vi "DataGraph_Facade.vi"(0 "Data In":T4, 2 "Display State In":T2, 3 "Container State":T3) -> (6 "Data Out":T4, 7 "Display State Out":T2, 8 "Action":T1)   [LabVIEW 2018, in "DataGraphXControl.xctl"]
uses:
  DataGraphXControl.xctl
  DataGraph_Data.ctl
  <vilib>/_xctls/Container State.ctl
  DataGraph_State.ctl
  <vilib>/_xctls/Action.ctl
  <vilib>/_xctls/XControlSupport.lvlib
panel:
  out "Title_Str":string
  in  "Output_Btn":bool
  in  "List_Btn":bool
  in  "Close_Btn":bool
  in  "Mark_Btn":bool
  out "Info_Listbox":i32(listbox)=-1
  out "Mass_Graph":cluster{"X":dbl[], "Y":dbl[]}[](graph)
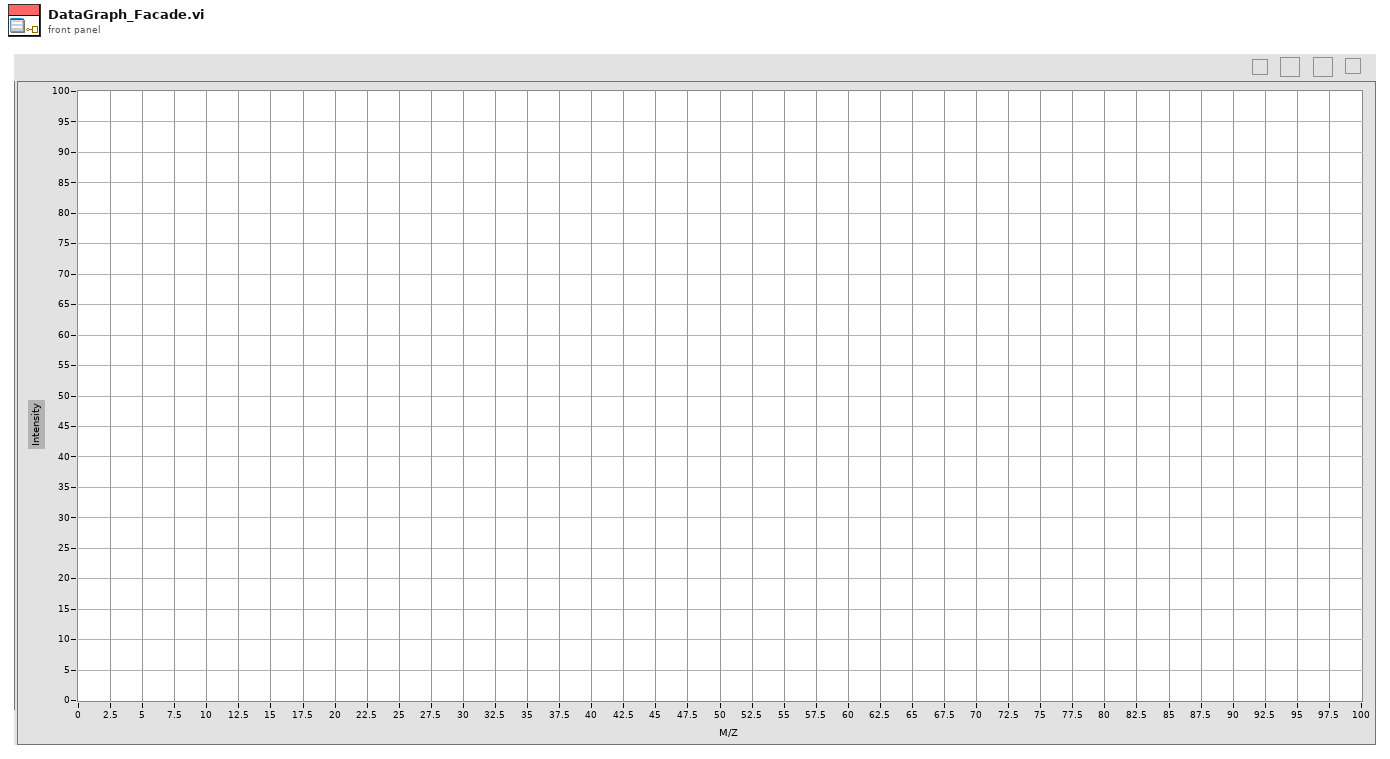
[diagram p1: front panel]
types:
  T1 = typedef "XControlSupport.lvlib/Action.ctl" = cluster{"Data Changed?":bool, "State Changed?":bool, "Action Name":string}
  T2 = typedef "DataGraphXControl.xctl/DataGraph_State.ctl" = cluster{"Mouse State":enum16{"Zoom In", "Select Range"}, "Rectangle X":cluster{"Minimum":dbl, "Maximum":dbl}, "Rectangle Y":cluster{"Minimum":dbl, "Maximum":dbl}, "X Index":cluster{"Minimum":u32, "Maximum":u32}, "FilePath":path, "Allow Index Bool":bool[], "Retangle Enable":bool, "Graph Enable":bool, "Aux Label Enable":bool}
  T3 = typedef "XControlSupport.lvlib/Container State.ctl" = cluster{"Indicator?":bool, "Run Mode?":bool, " Refnum":refnum<vi>}
  T4 = typedef "DataGraphXControl.xctl/DataGraph_Data.ctl" = cluster{"FilePath":path, "Data State":enum16{"Mass", "XIC"}, "Data Plot Names":string[], "DataArray":cluster{"X":dbl[], "Y":dbl[]}[], "Volt Plot Names":string[], "VoltArray":cluster{"X":dbl[], "Y":dbl[]}[], "UserDefine":cluster{"Label":string, "Variant":variant}, "Information":variant}
  T5 = enum16{"No Scaling", "Scale All Objects", "Scale Single Object"}
  T6 = enum8{"Enabled", "Disabled", "Disabled and Grayed Out"}
  T7 = typedef "LVRectTypeDef.ctl" = cluster{"Left":i16, "Top":i16, "Right":i16, "Bottom":i16}
  T8 = typedef "LVPoint32TypeDef.ctl" = cluster{"Horizontal":i32, "Vertical":i32}
  T9 = cluster{"X Scale.Range:Maximum":dbl, "X Scale.Range:Minimum":dbl, "Y Scale.Range:Maximum":dbl, "Y Scale.Range:Minimum":dbl}
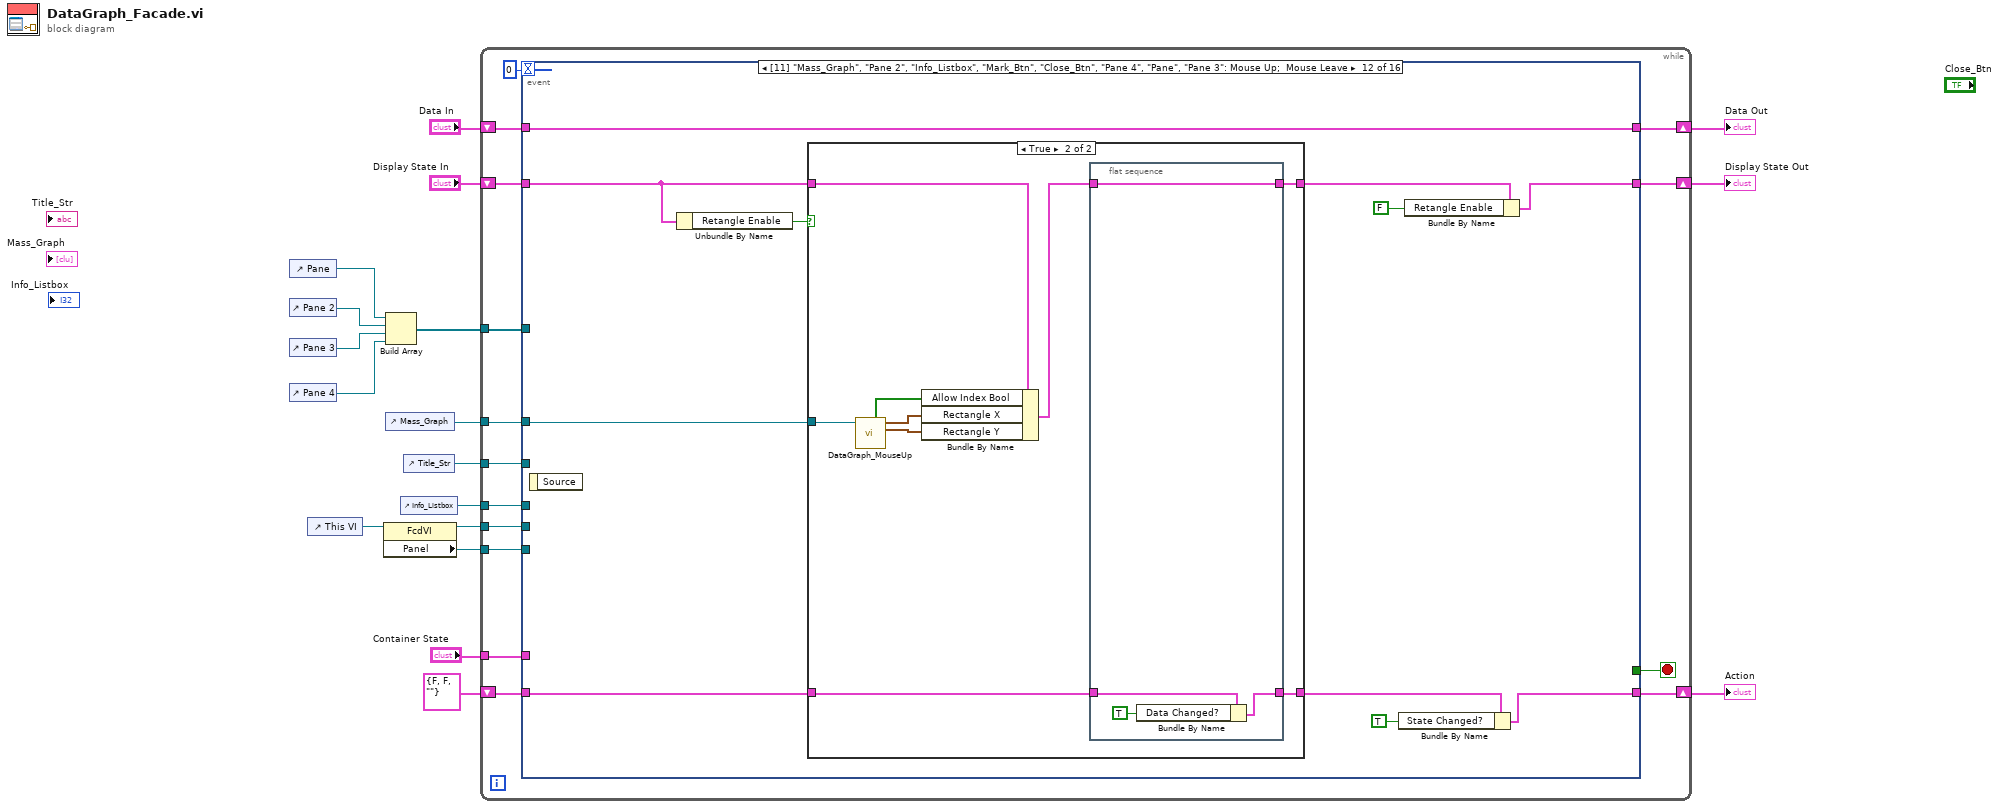
[diagram p0: block diagram]
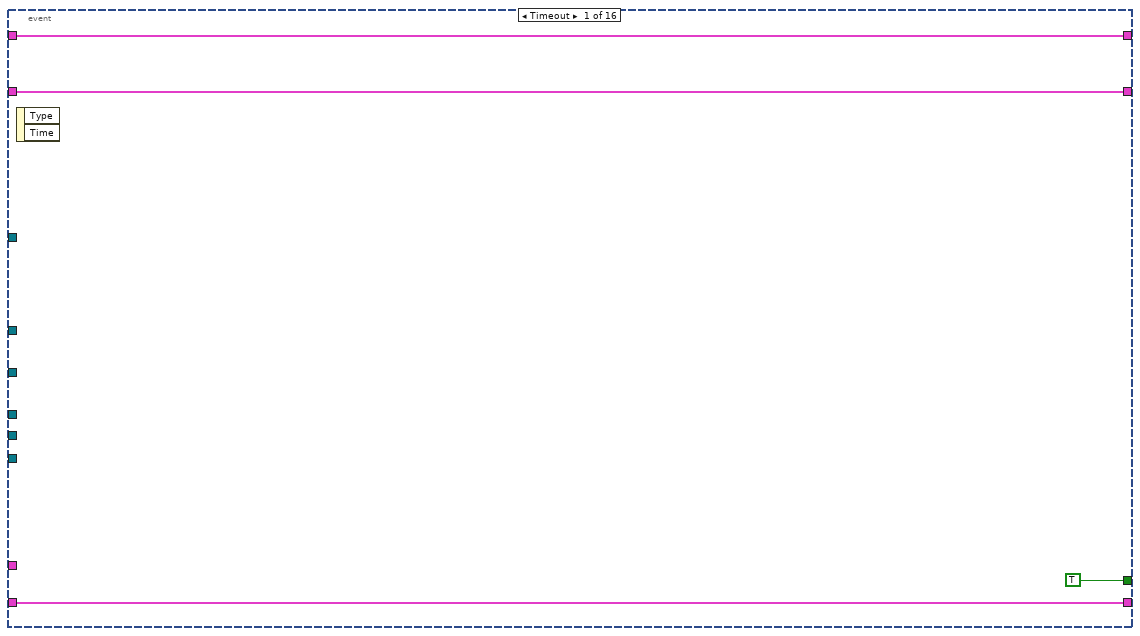
[diagram p2: hidden frame]
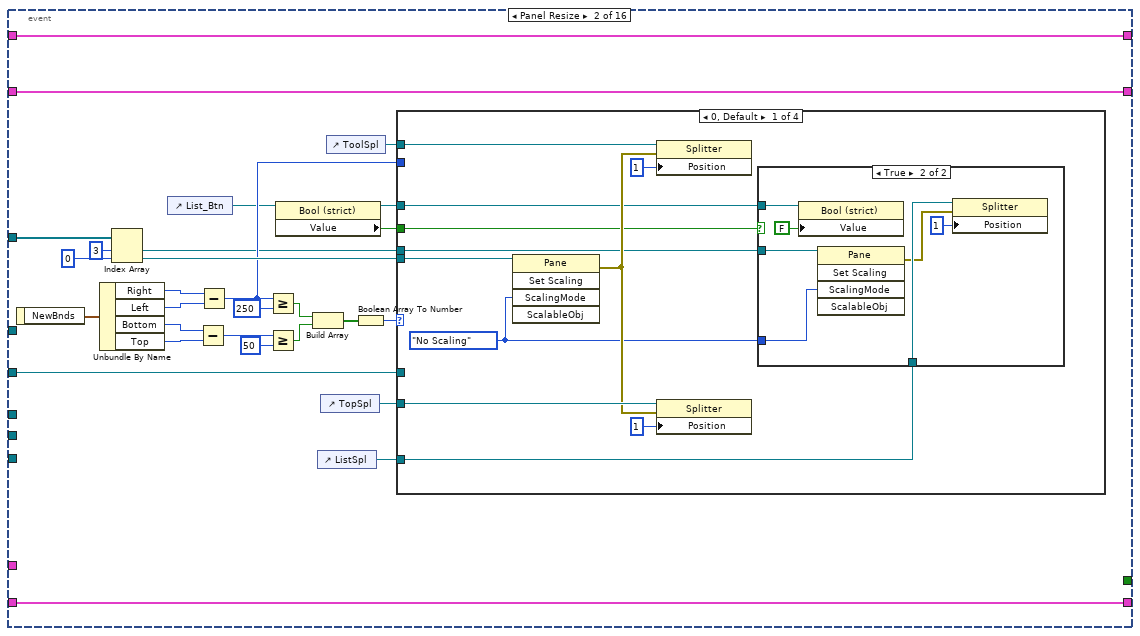
[diagram p3: hidden frame]
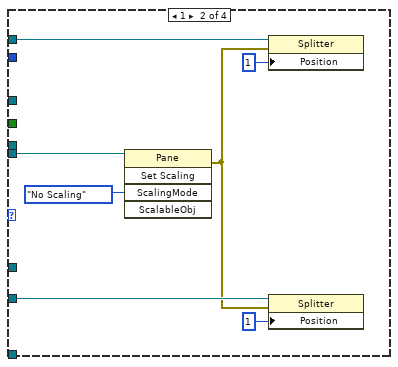
[diagram p5: hidden frame]
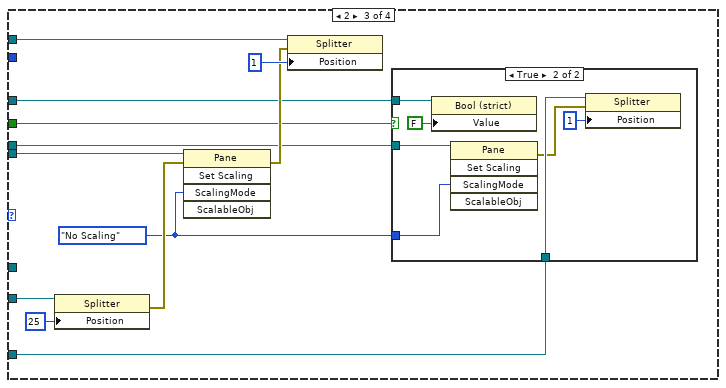
[diagram p6: hidden frame]
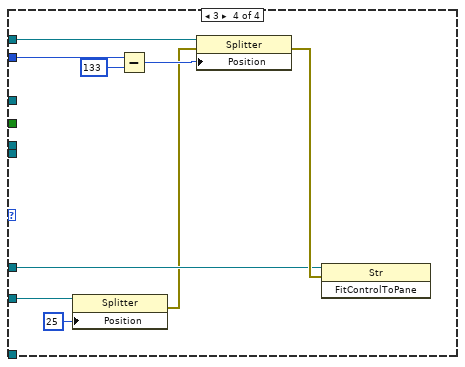
[diagram p8: hidden frame]
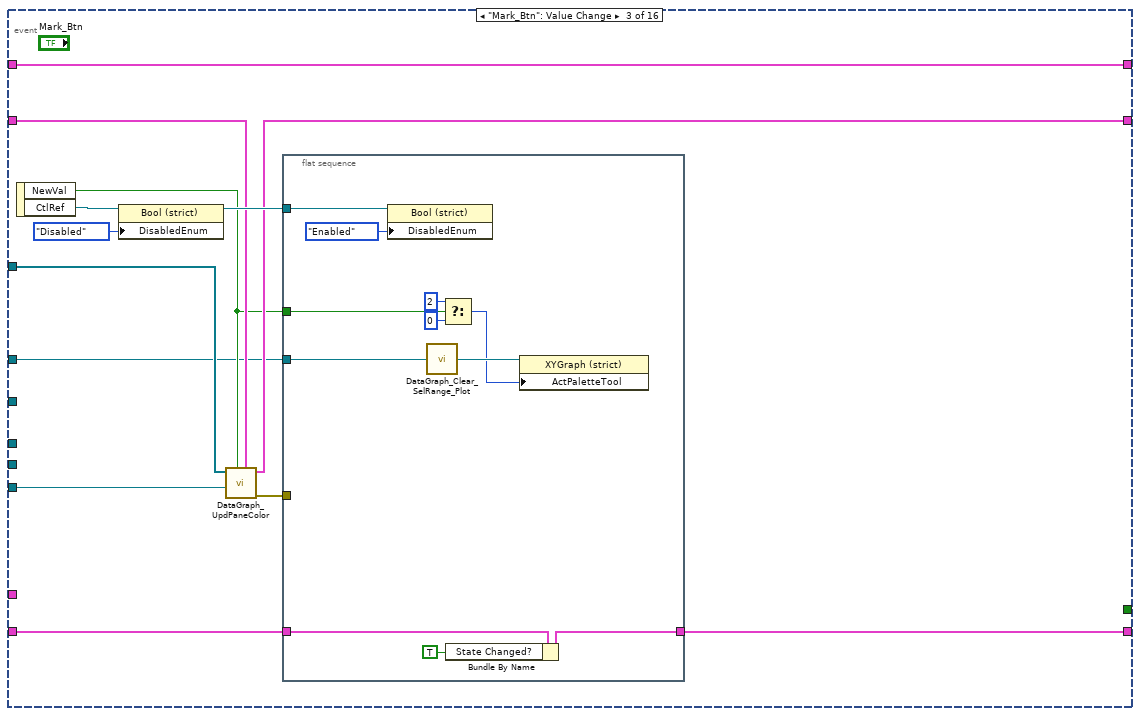
[diagram p9: hidden frame]
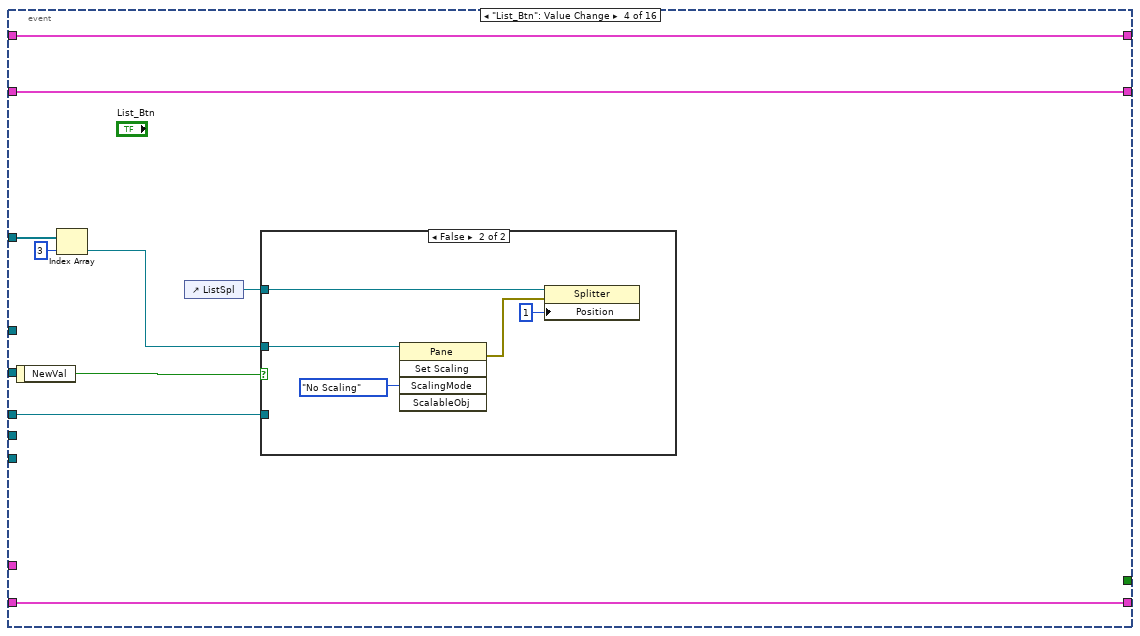
[diagram p10: hidden frame]
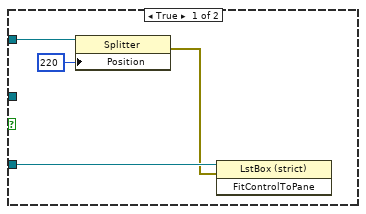
[diagram p11: hidden frame]
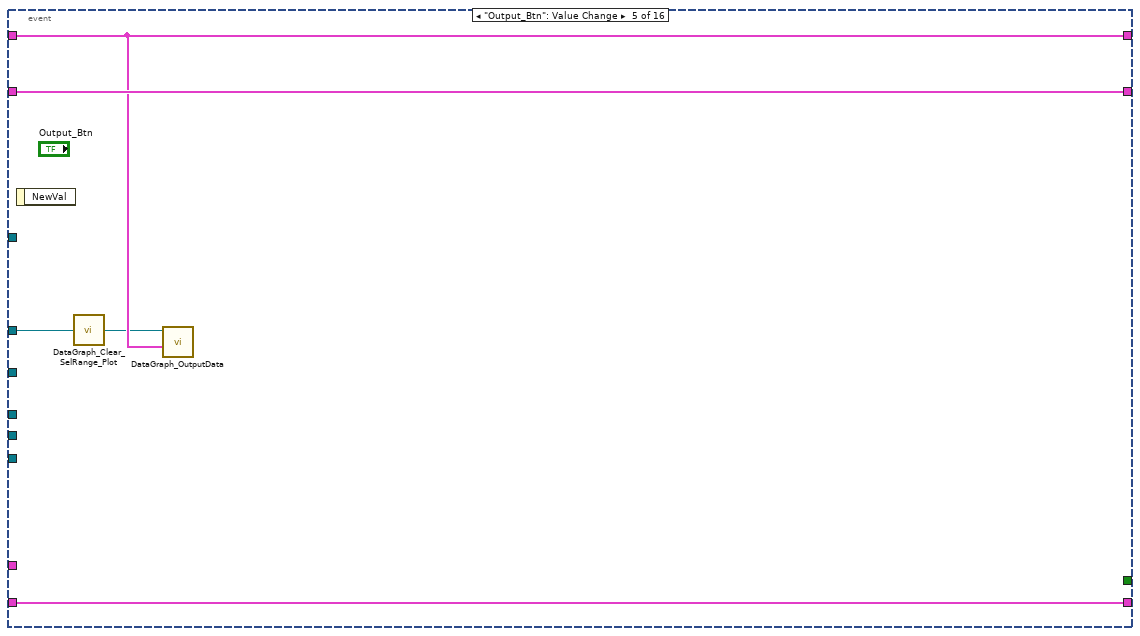
[diagram p12: hidden frame]
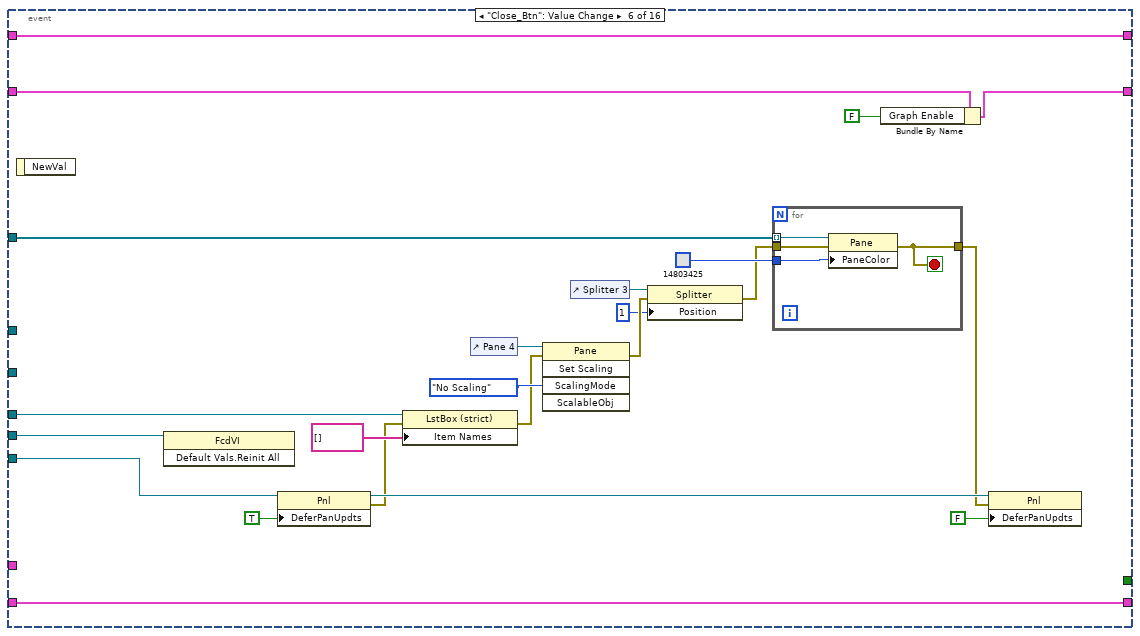
[diagram p13: hidden frame]
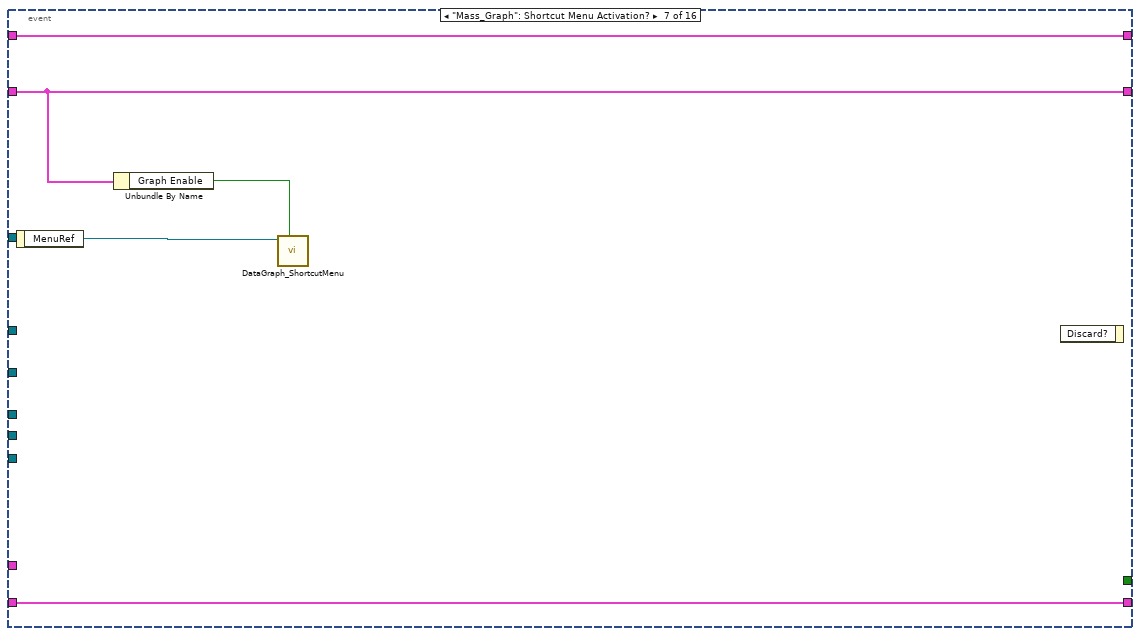
[diagram p14: hidden frame]
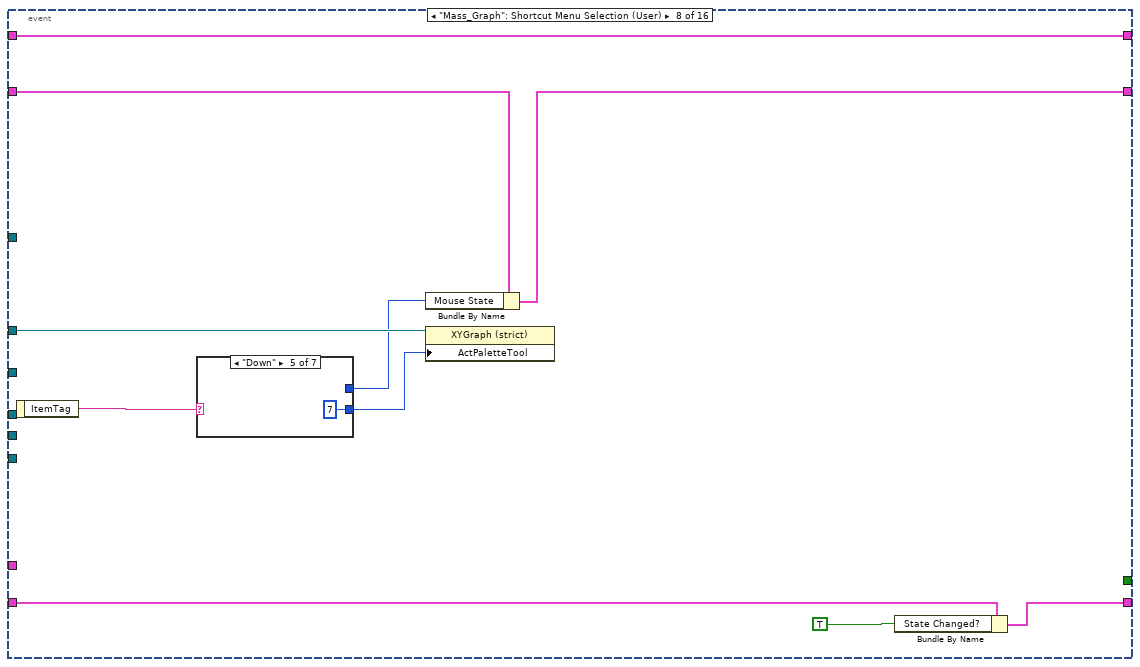
[diagram p15: hidden frame]
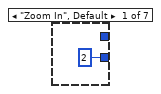
[diagram p16: hidden frame]
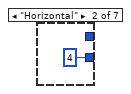
[diagram p17: hidden frame]
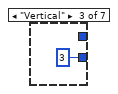
[diagram p18: hidden frame]
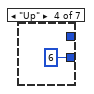
[diagram p19: hidden frame]
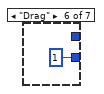
[diagram p20: hidden frame]
diagram:
  n1 = control-ref of="Pane"() -> (w5:refnum<vi>)
  n2 = control-ref of="Pane 2"() -> (w4:refnum<vi>)
  n3 = control-ref of="Pane 3"() -> (w3:refnum<vi>)
  n4 = control-ref of="Pane 4"() -> (w1:refnum<vi>)
  n5 = control-ref of="This VI"() -> (w8:refnum<vi>)
  n6 = property class="FcdVI"(reference=w8) -> (reference out=w6:refnum<vi>, "Panel"=w7:refnum<vi>)  [unwired: 1 in, 1 out]
  n7 = Build Array(w5, w4, w3, w1) -> (w2:refnum<vi>[])
  n8 = control-ref of="Mass_Graph"() -> (w11:refnum<vi>)
  n9 = control-ref of="Info_Listbox"() -> (w9:refnum<vi>)
  n10 = control-ref of="Title_Str"() -> (w10:refnum<vi>)
  n11 = while {
    shift-right: [w32] -> w15
    shift-left: "Display State In" -> [w33]
    tunnel: "Container State" -> [w29]
    shift-right: [w27] -> w18
    shift-left: "Data In" -> [w28]
    shift-right: [w25] -> w13
    shift-left: T1 {"Data Changed?"=FALSE, "State Changed?"=FALSE, "Action Name"=""} ("Action") -> [w26]
    tunnel: w11 -> [w24]
    tunnel: w10 -> [w23]
    tunnel: w9 -> [w22]
    tunnel: w7 -> [w21]
    tunnel: w6 -> [w20]
    tunnel: w2 -> [w19]
    stop <- w31 stop-if-true
    n12 = event shown="[11] \"Mass_Graph\", \"Pane 2\", \"Info_Listbox\", \"Mark_Btn\", \"Close_Btn\", \"Pane 4\", \"Pane\", \"Pane 3\": Mouse Up;  Mouse Leave" {
      selector: _ -> [_ _ _ _ _ _ _ _ _ _ _ _ _ _ _ _]
      dyn-events: _ -> [_ _ _ _ _ _ _ _ _ _ _ _ _ _ _ _]
      timeout: 0 -> [_ _ _ _ _ _ _ _ _ _ _ _ _ _ _ _]
      tunnel: w33 -> [w36 w65 w122 w151 w164 w177 w195 w202 w217 w245 w255 w275 w307 w313 w349 w353]
      tunnel: [w36 w65 w121 w151 w164 w176 w195 w201 w217 w244 w255 w272 w307 w312 w349 w353] -> w32
      tunnel: [TRUE _ _ _ _ _ _ _ _ _ _ _ _ _ _ _] -> w31
      tunnel: w29 -> [_ _ _ _ _ _ _ _ _ _ _ _ _ w321 w350 w354]
      tunnel: w28 -> [w35 w64 w131 w150 w163 w188 w197 w203 w224 w248 w258 w268 w305 w322 w348 w352]
      tunnel: [w35 w64 w131 w150 w163 w188 w197 w203 w224 w248 w258 w268 w305 w322 w348 w352] -> w27
      tunnel: [w34 w63 w129 w146 w165 w187 w196 w204 w223 w242 w257 w270 w306 w314 w347 w351] -> w25
      tunnel: w26 -> [w34 w63 w130 w146 w165 w187 w196 w205 w223 w243 w257 w266 w306 w315 w347 w351]
      tunnel: w24 -> [_ _ w119 _ w162 _ _ w207 w222 w241 _ w274 w302 w311 _ _]
      tunnel: w23 -> [_ w61 _ _ _ _ _ _ _ _ _ _ w303 _ _ _]
      tunnel: w22 -> [_ _ _ w147 _ w185 _ _ _ _ _ _ w304 _ _ _]
      tunnel: w21 -> [_ _ w127 _ _ w174 _ _ _ _ _ _ w296 w318 _ _]
      tunnel: w20 -> [_ _ _ _ _ w186 _ _ _ _ _ _ _ _ _ _]
      tunnel: w19 -> [_ w60 w128 w145 _ w178 _ _ _ _ _ _ _ w317 _ _]
      event Timeout {
        n13 = event-data() -> ()  [unwired: 1 in, 2 out]
      }
      event Panel Resize {
        n14 = event-data() -> ("NewBnds"=w48:T7)  [unwired: 1 in]
        n15 = Unbundle By Name(w48) -> ("Right"=w57:i16, "Left"=w56:i16, "Bottom"=w55:i16, "Top"=w54:i16)
        n16 = Index Array(array=w60, index #1=3 ("index"), index #2=0 ("index")) -> (element #1=w42:refnum<vi>, element #2=w58:refnum<vi>)
        n17 = control-ref of="List_Btn"() -> (w40:refnum<vi>)
        n18 = Subtract(x=w55, y=w54) -> (x-y=w52:i16)
        n19 = Subtract(x=w57, y=w56) -> (x-y=w45:i16)
        n20 = Greater Or Equal?(x=w45, y=i16 250) -> (x >= y?=w50:bool)
        n21 = Greater Or Equal?(x=w52, y=i16 50) -> (x >= y?=w49:bool)
        n22 = property class="Bool (strict)"(reference=w40) -> (reference out=w38:refnum<vi>, "Value"=w39:bool)  [unwired: 1 in, 1 out]
        n23 = Build Array(w50, w49) -> (w47:bool[])
        n24 = control-ref of="ListSpl"() -> (w41:refnum<vi>)
        n25 = control-ref of="TopSpl"() -> (w44:refnum<vi>)
        n26 = control-ref of="ToolSpl"() -> (w62:refnum<vi>)
        n27 = Boolean Array To Number(Boolean array=w47) -> (number=w46:u32)
        n28 = case shown="0, Default" w46 {
          tunnel: w62 -> [w76 w90 w97 w118]
          tunnel: w45 -> [_ _ _ w115]
          tunnel: w61 -> [_ _ _ w113]
          tunnel: w58 -> [w75 w89 w98 _]
          tunnel: w44 -> [w73 w86 w102 w111]
          tunnel: w42 -> [w70 _ w94 _]
          tunnel: w41 -> [w68 _ w93 _]
          tunnel: w39 -> [w67 _ w91 _]
          tunnel: w38 -> [w66 _ w92 _]
          frame 0, Default {
            w69 = T5."No Scaling" ("Scaling Mode")
            n29 = invoke class="Pane" method="Set Scaling"(reference=w75, "ScalingMode"=w69) -> (error out=w71:errorcluster)  [unwired: 3 in, 4 out]
            n30 = property class="Splitter"(reference=w76, error in=w71, "Position"=1 ("Splitter Position")) -> ()  [unwired: 2 out]
            n31 = property class="Splitter"(reference=w73, error in=w71, "Position"=1 ("Splitter Position")) -> ()  [unwired: 2 out]
            n32 = case shown="True" w67 {
              tunnel: w70 -> [_ w83]
              tunnel: w69 -> [_ w82]
              tunnel: w68 -> [_ w81]
              tunnel: w66 -> [_ w78]
              frame False {
              }
              frame True {
                n33 = property class="Bool (strict)"(reference=w78, "Value"=FALSE) -> ()  [unwired: 1 in, 2 out]
                n34 = invoke class="Pane" method="Set Scaling"(reference=w83, "ScalingMode"=w82) -> (error out=w79:errorcluster)  [unwired: 3 in, 4 out]
                n35 = property class="Splitter"(reference=w81, error in=w79, "Position"=1 ("Splitter Position")) -> ()  [unwired: 2 out]
              }
            }
          }
          frame 1 {
            n36 = invoke class="Pane" method="Set Scaling"(reference=w89, "ScalingMode"=T5."No Scaling" ("Scaling Mode")) -> (error out=w84:errorcluster)  [unwired: 3 in, 4 out]
            n37 = property class="Splitter"(reference=w90, error in=w84, "Position"=1 ("Splitter Position")) -> ()  [unwired: 2 out]
            n38 = property class="Splitter"(reference=w86, error in=w84, "Position"=1 ("Splitter Position")) -> ()  [unwired: 2 out]
          }
          frame 2 {
            w95 = T5."No Scaling" ("Scaling Mode")
            n39 = property class="Splitter"(reference=w102, "Position"=25 ("Splitter Position")) -> (error out=w96:errorcluster)  [unwired: 1 in, 1 out]
            n40 = invoke class="Pane" method="Set Scaling"(reference=w98, error in=w96, "ScalingMode"=w95) -> (error out=w99:errorcluster)  [unwired: 2 in, 4 out]
            n41 = property class="Splitter"(reference=w97, error in=w99, "Position"=1 ("Splitter Position")) -> ()  [unwired: 2 out]
            n42 = case shown="True" w91 {
              tunnel: w94 -> [_ w109]
              tunnel: w95 -> [_ w108]
              tunnel: w93 -> [_ w107]
              tunnel: w92 -> [_ w104]
              frame False {
              }
              frame True {
                n43 = property class="Bool (strict)"(reference=w104, "Value"=FALSE) -> ()  [unwired: 1 in, 2 out]
                n44 = invoke class="Pane" method="Set Scaling"(reference=w109, "ScalingMode"=w108) -> (error out=w105:errorcluster)  [unwired: 3 in, 4 out]
                n45 = property class="Splitter"(reference=w107, error in=w105, "Position"=1 ("Splitter Position")) -> ()  [unwired: 2 out]
              }
            }
          }
          frame 3 {
            n46 = property class="Splitter"(reference=w111, "Position"=25 ("Splitter Position")) -> (error out=w110:errorcluster)  [unwired: 1 in, 1 out]
            n47 = Subtract(x=w115, y=i16 133) -> (x-y=w116:i16)
            n48 = property class="Splitter"(reference=w118, error in=w110, "Position"=w116) -> (error out=w114:errorcluster)  [unwired: 1 out]
            n49 = invoke class="Str" method="FitControlToPane"(reference=w113, error in=w114) -> ()  [unwired: 1 in, 3 out]
          }
        }
      }
      event "Mark_Btn": Value Change {
        n50 = event-data() -> ("NewVal"=w120:bool, "CtlRef"=w125:refnum<vi>)  [unwired: 1 in]
        n51 = property class="Bool (strict)"(reference=w125, "DisabledEnum"=T6."Disabled" ("Disabled")) -> (reference out=w123:refnum<vi>)  [unwired: 1 in, 1 out]
        n52 = call "DataGraph_UpdPaneColor.vi"("Display State In"=w122, "Graph Enable"=w120, "Main VI Panel"=w127, "Pane Array"=w128) -> ("error out"=w126:errorcluster, "Display State Out"=w121:T2)  [unwired: 6 in]
        n53 = flat-sequence {
          tunnel: w130 -> [w142]
          tunnel: [w141] -> w129
          tunnel: w126 -> [_]
          tunnel: w123 -> [w138]
          tunnel: w120 -> [w135]
          tunnel: w119 -> [w134]
          frame #0 {
            n54 = property class="Bool (strict)"(reference=w138, "DisabledEnum"=T6."Enabled" ("Disabled")) -> ()  [unwired: 1 in, 2 out]
            n55 = call "DataGraph_Clear_SelRange_Plot.vi"("reference in"=w134) -> ("reference out"=w133:refnum<vi>)
            n56 = Select(t=2 ("Palette:Active Tool"), s=w135, f=0 ("Palette:Active Tool")) -> (s? t:f=w132:i32)
            n57 = Bundle By Name(cluster=w142, "State Changed?"=TRUE ("Data Changed?")) -> (w141:T1)
            n58 = property class="XYGraph (strict)"(reference=w133, "ActPaletteTool"=w132) -> ()  [unwired: 1 in, 2 out]
          }
        }
      }
      event "List_Btn": Value Change {
        n59 = event-data() -> ("NewVal"=w149:bool)  [unwired: 1 in]
        n60 = Index Array(array=w145, index=3) -> (element=w143:refnum<vi>)
        n61 = control-ref of="ListSpl"() -> (w148:refnum<vi>)
        n62 = case shown="False" w149 {
          tunnel: w148 -> [w154 w157]
          tunnel: w143 -> [_ w156]
          tunnel: w147 -> [w153 _]
          frame True {
            n63 = property class="Splitter"(reference=w154, "Position"=220 ("Splitter Position")) -> (error out=w152:errorcluster)  [unwired: 1 in, 1 out]
            n64 = invoke class="LstBox (strict)" method="FitControlToPane"(reference=w153, error in=w152) -> ()  [unwired: 1 in, 3 out]
          }
          frame False {
            n65 = invoke class="Pane" method="Set Scaling"(reference=w156, "ScalingMode"=T5."No Scaling" ("Scaling Mode")) -> (error out=w158:errorcluster)  [unwired: 3 in, 4 out]
            n66 = property class="Splitter"(reference=w157, error in=w158, "Position"=1 ("Splitter Position")) -> ()  [unwired: 2 out]
          }
        }
      }
      event "Output_Btn": Value Change {
        n67 = event-data() -> ()  [unwired: 1 in, 1 out]
        n68 = call "DataGraph_Clear_SelRange_Plot.vi"("reference in"=w162) -> ("reference out"=w161:refnum<vi>)
        n69 = call "DataGraph_OutputData.vi"("Data In"=w163, "Mass_Graph"=w161) -> ()  [unwired: 10 in]
      }
      event "Close_Btn": Value Change {
        n70 = event-data() -> ()  [unwired: 1 in, 1 out]
        n71 = invoke class="FcdVI" method="Default Vals.Reinit All"(reference=w186) -> ()  [unwired: 2 in, 3 out]
        n72 = property class="Pnl"(reference=w174, "DeferPanUpdts"=TRUE ("Defer Panel Updates")) -> (reference out=w182:refnum<vi>, error out=w167:errorcluster)  [unwired: 1 in]
        n73 = property class="LstBox (strict)"(reference=w185, error in=w167, "Item Names"=string[] []) -> (error out=w166:errorcluster)  [unwired: 1 out]
        n74 = control-ref of="Pane 4"() -> (w173:refnum<vi>)
        n75 = invoke class="Pane" method="Set Scaling"(reference=w173, error in=w166, "ScalingMode"=T5."No Scaling" ("Scaling Mode")) -> (error out=w171:errorcluster)  [unwired: 2 in, 4 out]
        n76 = control-ref of="Splitter 3"() -> (w172:refnum<vi>)
        n77 = property class="Splitter"(reference=w172, error in=w171, "Position"=1 ("Splitter Position")) -> (error out=w168:errorcluster)  [unwired: 1 out]
        n78 = for {
          tunnel: w178 -> [w192] mode=indexing
          tunnel: u32 14803425 -> [w191]
          tunnel: w168 -> [w190]
          tunnel: [w189] -> w179
          stop <- w189 stop-if-true
          n79 = property class="Pane"(reference=w192, error in=w190, "PaneColor"=w191) -> (error out=w189:errorcluster)  [unwired: 1 out]
        }
        n80 = Bundle By Name(cluster=w177, "Graph Enable"=FALSE) -> (w176:T2)
        n81 = property class="Pnl"(reference=w182, error in=w179, "DeferPanUpdts"=FALSE ("Defer Panel Updates")) -> ()  [unwired: 2 out]
      }
      event "Mass_Graph": Shortcut Menu Activation? {
        n82 = event-data() -> ("MenuRef"=w193:refnum<k9>)  [unwired: 1 in]
        n83 = Unbundle By Name(w195) -> ("Graph Enable"=w194:bool)
        n84 = call "DataGraph_ShortcutMenu.vi"("ShortCut Menu Enable"=w194, "menu reference"=w193) -> ()  [unwired: 8 in, 2 out]
        n85 = event-data() -> ()  [unwired: 2 in, 1 out]
      }
      event "Mass_Graph": Shortcut Menu Selection (User) {
        n86 = event-data() -> ("ItemTag"=w200:string)  [unwired: 1 in]
        n87 = case shown="\"Down\"" w200 {
          tunnel: [2 ("Palette:Active Tool") 4 ("Palette:Active Tool") 3 ("Palette:Active Tool") 6 ("Palette:Active Tool") 7 ("Palette:Active Tool") 1 ("Palette:Active Tool") 0 ("Palette:Active Tool")] -> w199
          tunnel: [_ _ _ _ _ _ enum16{"Zoom In", "Select Range"}."Select Range" ("Mouse State")] -> w198
          frame "Zoom In", Default {
          }
          frame "Horizontal" {
          }
          frame "Vertical" {
          }
          frame "Up" {
          }
          frame "Down" {
          }
          frame "Drag" {
          }
          frame "Select Range" {
          }
        }
        n88 = Bundle By Name(cluster=w202, "Mouse State"=w198) -> (w201:T2)
        n89 = property class="XYGraph (strict)"(reference=w207, "ActPaletteTool"=w199) -> ()  [unwired: 1 in, 2 out]
        n90 = Bundle By Name(cluster=w205, "State Changed?"=TRUE ("Data Changed?")) -> (w204:T1)
      }
      event "Mass_Graph": Mouse Down? {
        n91 = event-data() -> ("Button"=w221:u16, "Mods.Double Click"=w220:bool)  [unwired: 1 in]
        n92 = Unbundle By Name(w217) -> ("Mouse State"=w219:enum16{"Zoom In", "Select Range"})
        n93 = Equal?(x=w219, y=enum16{"Zoom In", "Select Range"}."Select Range") -> (x = y?=w216:bool)
        n94 = case shown="False" w216 {
          tunnel: w222 -> [w230 _]
          tunnel: w221 -> [w229 _]
          tunnel: w220 -> [w226 _]
          frame False {
            n95 = Equal?(x=u16 1, y=w229) -> (x = y?=w227:bool)
            n96 = And(x=w227, y=w226) -> (x .and. y?=w225:bool)
            n97 = case shown="True" w225 {
              tunnel: w230 -> [_ w231]
              frame False {
              }
              frame True {
                n98 = property class="XYGraph (strict)"(reference=w231, "ActPaletteTool"=5 ("Palette:Active Tool")) -> ()  [unwired: 1 in, 2 out]
              }
            }
          }
          frame True {
          }
        }
        n99 = event-data() -> ()  [unwired: 2 in, 1 out]
      }
      event "Mass_Graph": Mouse Down {
        n100 = event-data() -> ("Button"=w247:u16, "Coords"=w240:T8)  [unwired: 1 in]
        n101 = Unbundle By Name(w245) -> ("Mouse State"=w239:enum16{"Zoom In", "Select Range"})
        n102 = Equal?(x=u16 1, y=w247) -> (x = y?=w235:bool)
        n103 = Equal?(x=w239, y=enum16{"Zoom In", "Select Range"}."Select Range") -> (x = y?=w234:bool)
        n104 = And(x=w234, y=w235) -> (x .and. y?=w233:bool)
        n105 = case shown="True" w233 {
          selector: w233 -> [w249 w253]
          tunnel: w241 -> [_ w252]
          tunnel: [w249 w253] -> w237
          tunnel: w240 -> [_ w251]
          frame False {
          }
          frame True {
            n106 = call "DataGraph_MouseInit.vi"("State"=enum16{"Read", "Write"}."Write", "Point32"=w251, "Mass_Graph"=w252) -> ()  [unwired: 5 in, 4 out]
          }
        }
        n107 = Bundle By Name(cluster=w243, "State Changed?"=TRUE) -> (w242:T1)
        n108 = Bundle By Name(cluster=w245, "Retangle Enable"=w237) -> (w244:T2)
      }
      event "Mass_Graph": Mouse Move {
        n109 = event-data() -> ("Coords"=w256:T8)  [unwired: 1 in]
        n110 = Unbundle By Name(w255) -> ("Retangle Enable"=w254:bool)
        n111 = case shown="True" w254 {
          tunnel: w256 -> [_ w260]
          frame False {
          }
          frame True {
            n112 = call "DataGraph_MouseInit.vi"("State"=enum16{"Read", "Write"}."Read") -> ("error out"=w264:errorcluster, "Point32"=w262:T8, "reference out"=w263:refnum<vi>, "Boundary"=w259:T9)  [unwired: 7 in]
            n113 = call "DataGraph_MouseMove.vi"("Boundary"=w259, "error in (no error)"=w264, "Point32"=w260, "Raw Coords"=w262, "Mass_Graph"=w263) -> ()  [unwired: 6 in, 1 out]
          }
        }
      }
      event "Mass_Graph", "Info_Listbox", "Mark_Btn", "Close_Btn": Mouse Up; Mouse Leave {
        n114 = event-data() -> ()  [unwired: 1 in, 1 out]
        n115 = Unbundle By Name(w275) -> ("Retangle Enable"=w273:bool)
        n116 = case shown="True" w273 {
          tunnel: w275 -> [w277 w286]
          tunnel: w274 -> [_ w285]
          tunnel: [w277 w282] -> w269
          tunnel: w266 -> [w276 w284]
          tunnel: [w276 w283] -> w265
          frame False {
          }
          frame True {
            n117 = call "DataGraph_MouseUp.vi"("Mass_Graph"=w285) -> ("Rectangle Y"=w279:cluster{"Minimum":dbl, "Maximum":dbl}, "Rectangle X"=w280:cluster{"Minimum":dbl, "Maximum":dbl}, "Allow Index Bool"=w278:bool[])  [unwired: 7 in, 1 out]
            n118 = Bundle By Name(cluster=w286, "Allow Index Bool"=w278, "Rectangle X"=w280, "Rectangle Y"=w279) -> (w281:T2)
            n119 = flat-sequence {
              tunnel: w284 -> [w290]
              tunnel: [w288] -> w283
              tunnel: [w287] -> w282
              tunnel: w281 -> [w287]
              frame #0 {
                n120 = Bundle By Name(cluster=w290, "Data Changed?"=TRUE) -> (w288:T1)
              }
            }
          }
        }
        n121 = Bundle By Name(cluster=w265, "State Changed?"=TRUE) -> (w270:T1)
        n122 = Bundle By Name(cluster=w269, "Retangle Enable"=FALSE) -> (w272:T2)
      }
      event Data Change {
        n123 = event-data() -> ()  [unwired: 1 in, 1 out]
        n124 = property class="Pnl"(reference=w296, "DeferPanUpdts"=TRUE ("Defer Panel Updates")) -> (reference out=w292:refnum<vi>, error out=w294:errorcluster)  [unwired: 1 in]
        n125 = call "DataGraph_UpdateInterface.vi"("Data In"=w305, "error in (no error)"=w294, "Info_Listbox"=w304, "Title_Str"=w303, "Mass_Graph"=w302) -> ("error out"=w301:errorcluster)  [unwired: 6 in]
        n126 = property class="XYGraph (strict)"(reference=w302, error in=w301, "ActPaletteTool"=0 ("Palette:Active Tool")) -> (reference out=w299:refnum<vi>, error out=w298:errorcluster)
        n127 = property class="XYGraph (strict)"(reference=w299, error in=w298, "ActPaletteTool"=5 ("Palette:Active Tool")) -> (error out=w291:errorcluster)  [unwired: 1 out]
        n128 = property class="Pnl"(reference=w292, error in=w291, "DeferPanUpdts"=FALSE ("Defer Panel Updates")) -> ()  [unwired: 2 out]
      }
      event Display State Change {
        n129 = event-data() -> ()  [unwired: 1 in, 1 out]
        n130 = Unbundle By Name(w313) -> ("Aux Label Enable"=w309:bool, "Graph Enable"=w319:bool)
        n131 = Unbundle By Name(w321) -> ("Run Mode?"=w320:bool)
        n132 = case shown="True" w320 {
          tunnel: w319 -> [_ w340]
          tunnel: w318 -> [_ w345]
          tunnel: w317 -> [_ w346]
          tunnel: w313 -> [w333 w343]
          tunnel: [w333 w342] -> w312
          tunnel: w311 -> [w332 w341]
          tunnel: [w332 w335] -> w310
          tunnel: w309 -> [w331 w334]
          tunnel: [w331 w334] -> w308
          frame False {
          }
          frame True {
            n133 = call "DataGraph_UpdPaneColor.vi"("Display State In"=w343, "Graph Enable"=w340, "Main VI Panel"=w345, "Pane Array"=w346) -> ("error out"=w344:errorcluster, "Display State Out"=w342:T2)  [unwired: 6 in]
            n134 = property on="Mark_Btn" class="Bool (strict)"(error in=w344, "Value"=w340) -> (error out=w336:errorcluster)  [unwired: 1 in, 1 out]
            n135 = Select(t=2 ("Palette:Active Tool"), s=w340, f=0 ("Palette:Active Tool")) -> (s? t:f=w338:i32)
            n136 = property class="XYGraph (strict)"(reference=w341, error in=w336, "ActPaletteTool"=w338) -> (reference out=w335:refnum<vi>)  [unwired: 1 out]
          }
        }
        n137 = case shown="False" w308 {
          tunnel: w310 -> [w326 w330]
          frame True {
            n138 = property class="XYGraph (strict)"(reference=w326, "ActYScl"=1 ("Active Y Scale")) -> (reference out=w324:refnum<vi>)  [unwired: 1 in, 1 out]
            n139 = property class="XYGraph (strict)"(reference=w324, "YScale.Style"=u8 0 ("Y Scale.Style")) -> ()  [unwired: 1 in, 2 out]
          }
          frame False {
            n140 = property class="XYGraph (strict)"(reference=w330, "ActYScl"=1 ("Active Y Scale")) -> (reference out=w328:refnum<vi>)  [unwired: 1 in, 1 out]
            n141 = property class="XYGraph (strict)"(reference=w328, "YScale.Style"=u8 5 ("Y Scale.Style")) -> ()  [unwired: 1 in, 2 out]
          }
        }
        n142 = Bundle By Name(cluster=w315, "State Changed?"=TRUE) -> (w314:T1)
      }
      event Direction Change {
        n143 = event-data() -> ()  [unwired: 1 in, 1 out]
        n144 = Unbundle By Name(w350) -> ()  [unwired: 1 out]
      }
      event Exec State Change {
        n145 = event-data() -> ()  [unwired: 1 in, 1 out]
        n146 = Unbundle By Name(w354) -> ()  [unwired: 1 out]
      }
    }
  }
  "Display State Out" <- w15
  "Data Out" <- w18
  "Action" <- w13
